vi "Rotations to Degrees.vi"(11 "rotations":dbl) -> (3 "degrees":dbl)   [LabVIEW 2020]
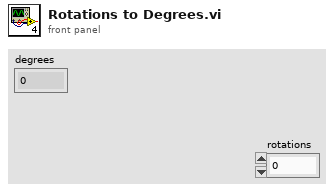
[diagram p1: front panel]
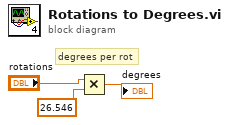
[diagram p0: block diagram]
diagram:
  # "degrees per rot"
  n1 = Multiply(x="rotations", y=26.546) -> (x*y=→"degrees":dbl)
